vi "CoMP-S TDMS for Camera.vi"(6 "HandleOut":u32, 7 "Input h":u64, 8 "hout SetRec":u64, 9 "h buffer":u64, 10 "GetRecState":u16, 11 "SerialNumber":u32) -> (2 "TDMS Cams Output":string[][](array[string]), 3 "TDMS Channel Name":string[](array[string]))   [LabVIEW 2014]
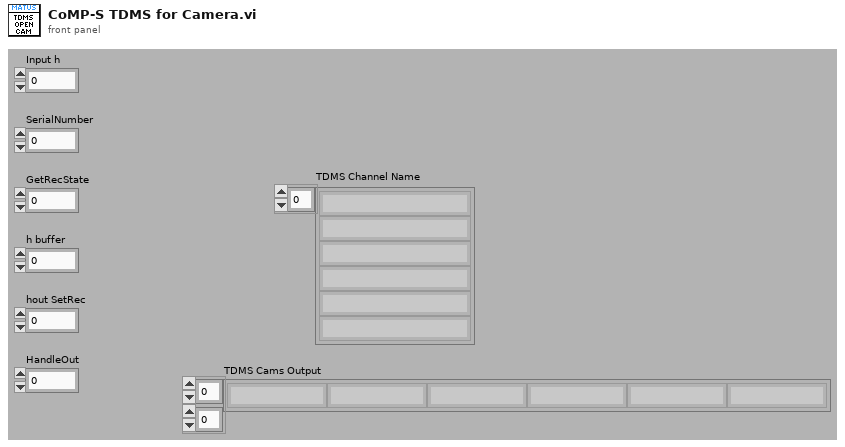
[diagram p1: front panel]
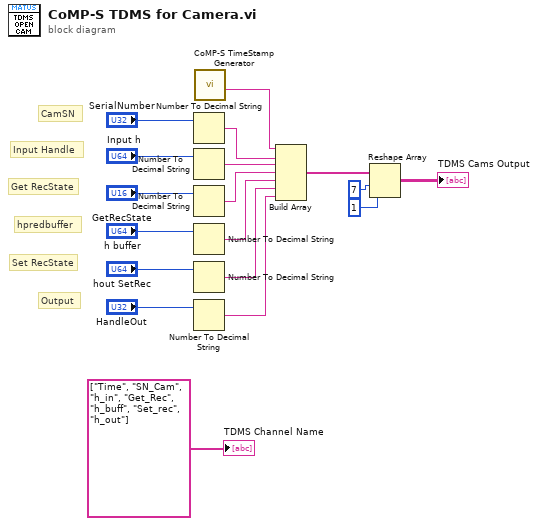
[diagram p0: block diagram]
diagram:
  # "hpredbuffer"
  # "CamSN"
  # "Input Handle"
  # "Get RecState"
  # "Output"
  # "Set RecState"
  n1 = Number To Decimal String(number="SerialNumber") -> (decimal integer string=w13:string)  [unwired: 1 in]
  n2 = Number To Decimal String(number="Input h") -> (decimal integer string=w14:string)  [unwired: 1 in]
  n3 = Number To Decimal String(number="GetRecState") -> (decimal integer string=w15:string)  [unwired: 1 in]
  n4 = Number To Decimal String(number="h buffer") -> (decimal integer string=w16:string)  [unwired: 1 in]
  n5 = Number To Decimal String(number="hout SetRec") -> (decimal integer string=w17:string)  [unwired: 1 in]
  n6 = Number To Decimal String(number="HandleOut") -> (decimal integer string=w18:string)  [unwired: 1 in]
  n7 = call "CoMP-S TimeStamp Generator.vi"() -> ("date/time string"=w1:string)  [unwired: 10 in, 1 out]
  n8 = Build Array(w1, w13, w14, w15, w16, w17, w18) -> (w6:string[])
  n9 = Reshape Array(w6, 7 ("dimension size"), 1 ("dimension size")) -> (→"TDMS Cams Output":string[][])
  "TDMS Channel Name" <- string[] ["Time", "SN_Cam", "h_in", "Get_Rec", "h_buff", "Set_rec", "h_out"] ("Channel Name")
